vi "TW Post-Project-Copying Process - Stage 3.vi"(8 "error in":errorcluster, 10 "Project Name":string, 11 "User Project Path":path) -> (0 "error out":errorcluster)   [LabVIEW 2021, in "Plugin Generator.lvlib"]
uses:
  Plugin Generator.lvlib
  Typedef/Plugin OS.ctl
  <vilib>/Utility/EditLVProj/Edit LVProj.lvlib
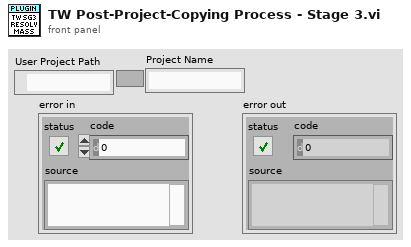
[diagram p1: front panel]
types:
  T1 = typedef "Plugin Generator.lvlib/Plugin OS.ctl" = enum16{"Linux RT", "Env Server"}
  T2 = typedef "Edit LVProj.lvlib/Library And VI References.ctl" = cluster{"Target Reference":refnum<vi>, "VI References":refnum<vi>[], "Library References":refnum<vi>[]}
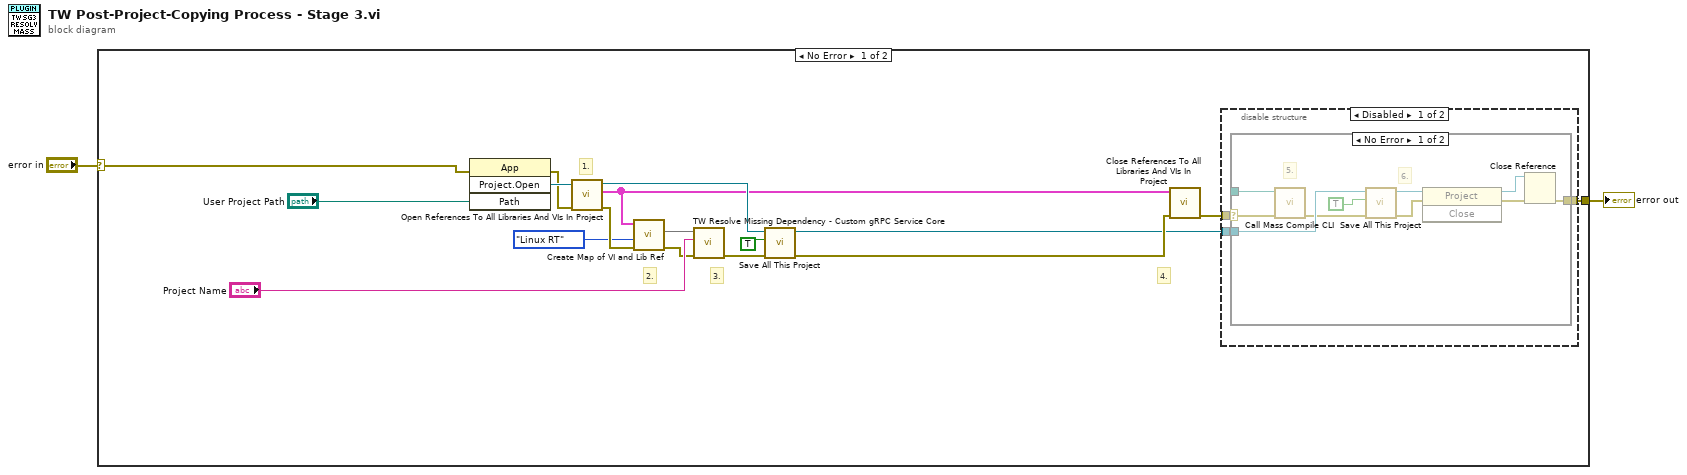
[diagram p0: block diagram]
diagram:
  n1 = case shown="No Error" "error in" {
    selector: "error in" -> [w8 w35]
    tunnel: [w19 w35] -> w2
    frame No Error {
      # "4."
      # "3."
      # "2."
      # "1."
      n2 = invoke class="App" method="Project.Open"(error in=w8, "Path"="User Project Path") -> (error out=w17:errorcluster, "Project:Open"=w18:refnum<vi>)  [unwired: 2 in, 2 out]
      n3 = call <vilib>:"Open References To All Libraries And VIs In Project.vi"("error in (no error)"=w17, "Project in"=w18) -> ("error out"=w11:errorcluster, "VI and Library References"=w13:T2[], "Project out"=w15:refnum<vi>)  [unwired: 7 in]
      n4 = call "Create Map of VI and Lib Ref.vi"("error in"=w11, "Plugin OS"=Plugin_OS."Linux RT", "VI and Library References"=w13) -> ("error out"=w4:errorcluster, "Map - LibRef"=w6:map{string, refnum<vi>})  [unwired: 6 in, 1 out]
      n5 = call "TW Resolve Missing Dependency - Custom gRPC Service Core.vi"("error in"=w4, "Project Name"="Project Name", "Map - LibRef"=w6) -> ("error out"=w3:errorcluster)  [unwired: 8 in]
      n6 = call <vilib>:"Save All This Project.vi"("error in (no error)"=w3, "Exclude Dependencies? (F)"=TRUE, "Project in"=w15) -> ("error out"=w14:errorcluster, "Project out"=w12:refnum<vi>)  [unwired: 7 in]
      n7 = call <vilib>:"Close References To All Libraries And VIs In Project.vi"("error in (no error)"=w14, "VI and Library References"=w13) -> ("error out"=w10:errorcluster)  [unwired: 9 in]
      n8 = disable-structure shown="Disabled" {
        disable-tunnel: [w22 w34] -> w19
        disable-tunnel: w12 -> [w21 _]
        disable-tunnel: w10 -> [w20 w34]
        frame Disabled {
          n9 = case shown="No Error" w20 {
            selector: w20 -> [w23 w33]
            tunnel: [w32 w33] -> w22
            tunnel: w21 -> [w28 _]
            tunnel: _ -> [w24 _]
            frame No Error {
              # "6."
              # "5."
              n10 = call "Call Mass Compile CLI.vi"("error in"=w23, "Project Root"=w24) -> ("error out"=w25:errorcluster)  [unwired: 9 in]
              n11 = call <vilib>:"Save All This Project.vi"("error in (no error)"=w25, "Exclude Dependencies? (F)"=TRUE, "Project in"=w28) -> ("error out"=w29:errorcluster, "Project out"=w30:refnum<vi>)  [unwired: 7 in]
              n12 = invoke class="Project" method="Close"(reference=w30, error in=w29) -> (reference out=w27:refnum<vi>, error out=w26:errorcluster)  [unwired: 1 in, 1 out]
              n13 = Close Reference(reference=w27, error in (no error)=w26) -> (error out=w32:errorcluster)
            }
            frame Error {
            }
          }
        }
        frame Enabled {
        }
      }
    }
    frame Error {
    }
  }
  "error out" <- w2
